vi "Send Exit.vi"(8 "error in (no error)":errorcluster, 11 "qbus in":refnum<class "Qbus.lvclass">) -> (0 "error out":errorcluster, 3 "qbus out":refnum<class "Qbus.lvclass">)   [LabVIEW 2015, in "Exposure Process.lvlib"]
doc: "Registers an event with the Timer process. When the event timer expires, the timer sends the callback action and value to the specified process."
uses:
  Exposure Process.lvlib
  <vilib>/addons/Qbus/Qbus.lvclass
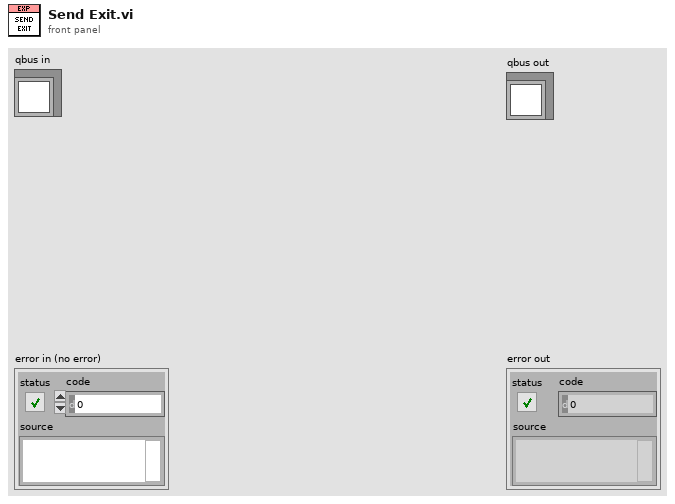
[diagram p1: front panel]
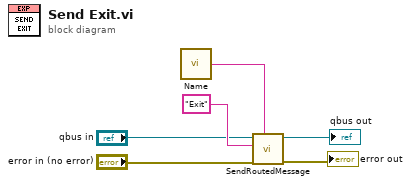
[diagram p0: block diagram]
diagram:
  n1 = call "Name.vi"() -> ("process name"=w4:string)  [unwired: 5 in]
  n2 = call <vilib>:"SendRoutedMessage.vi"("listener process"=w4, "error in (no error)"="error in (no error)", "message name"="Exit" ("MsgName"), "Qbus in"="qbus in") -> ("error in (no error)"=→"error out":errorcluster, "Qbus out"=→"qbus out":refnum<class "Qbus.lvclass">)  [unwired: 6 in]
